vi "ReadCoord.vi"(8 "error in (no error)":errorcluster, 10 "Engine":dbl, 11 "connection ID":refnum<k16>) -> (0 "error out (no error)":errorcluster, 1 "X":dbl, 2 "Y":dbl, 3 "connection ID out":refnum<k16>, 7 "error out":errorcluster)   [LabVIEW 2019]
panel:
  in  "Stop":bool
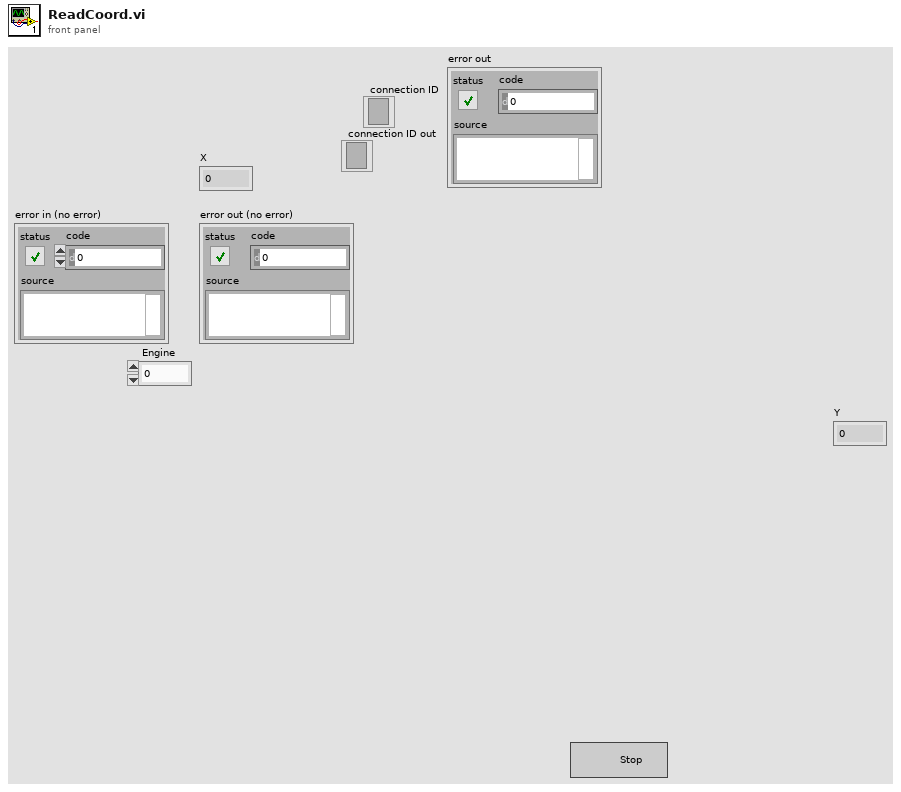
[diagram p1: front panel]
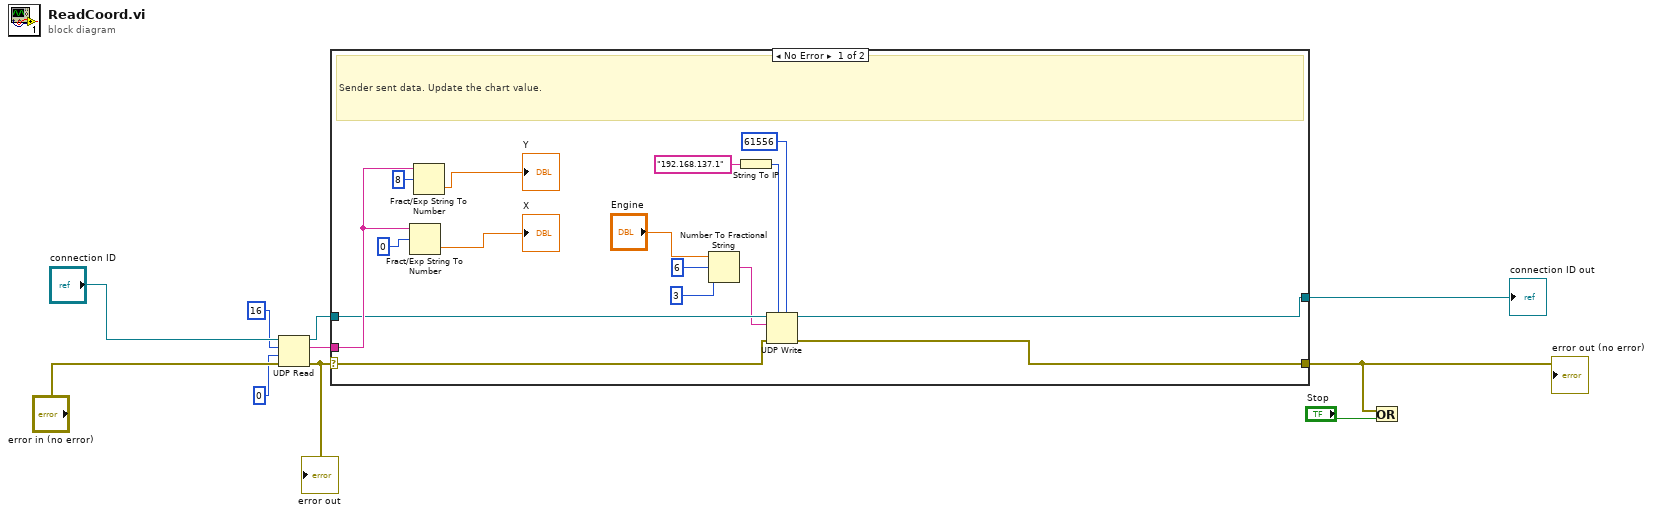
[diagram p0: block diagram]
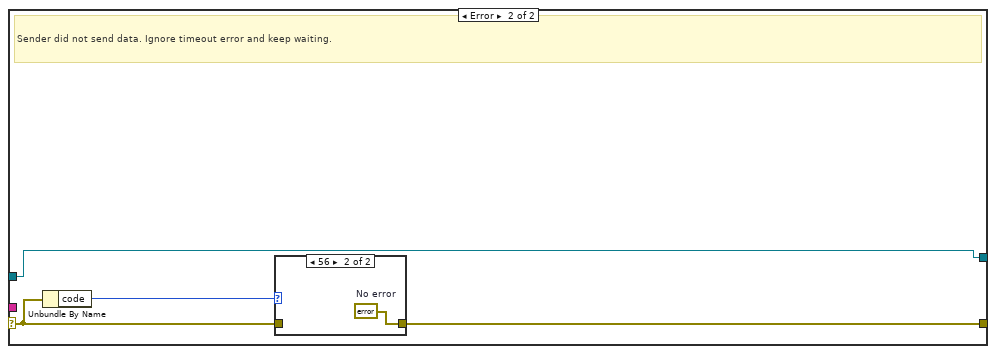
[diagram p2: hidden frame]
diagram:
  n1 = UDP Read(connection ID="connection ID", max size (548)=16, timeout ms (25000)=0, 8:"error in (no error)") -> (data out=w5:string, error out=w4:errorcluster, 3:w2:refnum<k16>)  [unwired: 2 out]
  "error out" <- w4
  n2 = case shown="No Error" w4 {
    selector: w4 -> [w17 w29]
    tunnel: w5 -> [w24 _]
    tunnel: [w11 w28] -> w10
    tunnel: w2 -> [w18 w27]
    tunnel: [w12 w27] -> w1
    frame No Error {
      # "Sender sent data. Update the chart value."
      n3 = Fract/Exp String To Number(string=w24, offset=0) -> (number=→"X":dbl)  [unwired: 2 in, 1 out]
      n4 = Fract/Exp String To Number(string=w24, offset=8) -> (number=→"Y":dbl)  [unwired: 2 in, 1 out]
      n5 = Number To Fractional String(number="Engine", width (-)=i16 6, precision (6)=i16 3) -> (F-format string=w15:string)  [unwired: 1 in]
      n6 = String To IP(1:"192.168.137.1" ("name")) -> (0:w20:u32)
      n7 = UDP Write(address=w20, port or service name=u16 61556, connection ID=w18, data in=w15, 8:w17) -> (error out=w11:errorcluster, 3:w12:refnum<k16>)  [unwired: 1 in]
    }
    frame Error {
      # "Sender did not send data. Ignore timeout error and keep waiting."
      n8 = Unbundle By Name(w29) -> ("code"=w30:i32)
      n9 = case shown="56" w30 {
        tunnel: w29 -> [w31 _]
        tunnel: [w31 w32] -> w28
        frame Default {
        }
        frame 56 {
          w32 = errorcluster {"status"=FALSE, "code"=0, "source"=""}  # No error
        }
      }
    }
  }
  "error out (no error)" <- w10
  "connection ID out" <- w1
  n10 = Or(x=w10, y="Stop") -> ()  [unwired: 1 out]
